vi "Test_API_InitInvalidInput_NoLogger.vi"(8 "error in (no error)":errorcluster, 11 "TestCase in":refnum<class "TestLocalLogInstance.lvclass">) -> (0 "error out":errorcluster, 3 "TestCase out":refnum<class "TestLocalLogInstance.lvclass">)   [LabVIEW 2017, in "TestLocalLogInstance.lvclass"]
uses:
  TestLocalLogInstance.lvclass
  Source/Composed Log/LoggerReference/LoggerReference.lvclass/LoggerReference.ctl
  9a0b009a-159a-478b-8bd0-efcaa49947a6.vi
  Source/Composed Log/LoggerReference/Return Aggregate Queues.vi
  Source/Composed Log/LoggerReference/Add Aggregate Log.vi
  9a0b009a-159a-478b-8bd0-efcaa49947a6.vi/c08b9aa3-6762-45d9-a18e-2ba9e4946dcb.vi
  Source/Composed Log/LoggerReference/Log.vi
  Source/Composed Log/LoggerReference/Send Add Sink.vi
  Source/Composed Log/LoggerReference/Remove Stale Logs.vi
  Source/Composed Log/Application Logger/Launch Worker Loop.vi
  Source/Composed Log/LoggerReference/Initialize Logger Instance.vi
  Source/Composed Log/Log Sink/Log Sink.lvclass
  Source/Composed Log/LoggerReference/LoggerReference.lvclass
  Source/Composed Log/IErrorFormat/IErrorFormat.lvclass
  <vilib>/addons/_JKI Toolkits/VI Tester/TestCase.llb/TestCase.lvclass
  C:/Program Files (x86)/National Instruments/LabVIEW 2017/vi.lib/addons/_JKI Toolkits/VI Tester/TestCase.llb/TestCase.lvclass
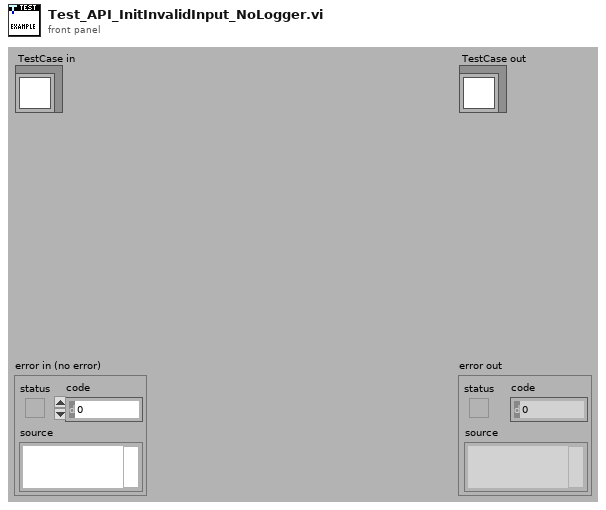
[diagram p1: front panel]
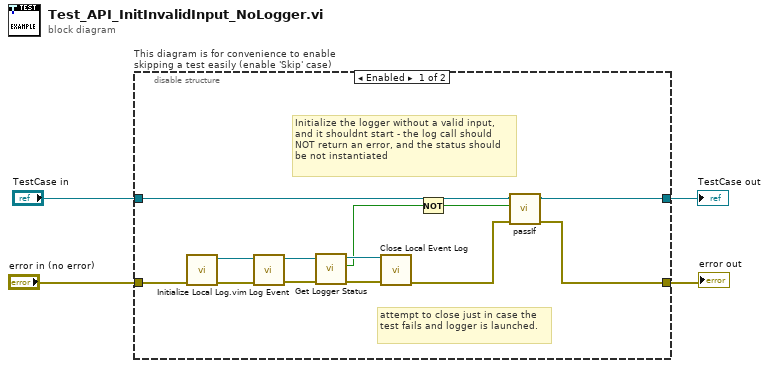
[diagram p0: block diagram]
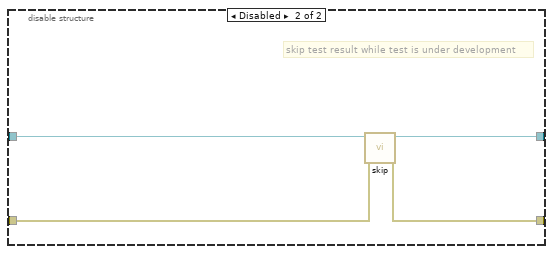
[diagram p2: hidden frame]
diagram:
  n1 = disable-structure "This diagram is for convenience to enable skipping a test easily (enable 'Skip' case)" shown="Enabled" {
    disable-tunnel: "TestCase in" -> [w14 w21]
    disable-tunnel: [w12 w19] -> w1
    disable-tunnel: [w11 w20] -> w3
    disable-tunnel: "error in (no error)" -> [w17 w18]
    frame Enabled {
      # "attempt to close just in case the test fails and logger is launched."
      # "Initialize the logger without a valid input, and it shouldnt start - the log call should  NOT return an error, and the status should be not instantiated"
      n2 = call "Initialize Local Log.vim"("error in (no error)"=w17) -> ("error out"=w16:errorcluster, "Log Instance Reference"=w15:refnum<class "LoggerReference.lvclass">)  [unwired: 8 in, 1 out]
      n3 = call "Log Event.vi"("error in (no error)"=w16, "Log Instance"=w15) -> ("error out"=w9:errorcluster, "Log Instance Out"=w10:refnum<class "LoggerReference.lvclass">)  [unwired: 8 in]
      n4 = call "Get Logger Status.vi"("error in (no error)"=w9, "LoggerReference in"=w10) -> ("error out"=w8:errorcluster, "Logger Instantiated?"=w6:bool, "LoggerReference out"=w7:refnum<class "LoggerReference.lvclass">)  [unwired: 6 in, 1 out]
      n5 = call "Close Local Event Log.vi"("error in (no error)"=w8, "Log Instance"=w7) -> ("error out"=w13:errorcluster)  [unwired: 9 in]
      n6 = Not(x=w6) -> (.not. x?=w5:bool)
      n7 = call-dynamic "passIf.vi"("error in (no error)"=w13, "pass"=w5, "TestCase in"=w14) -> ("error out"=w11:errorcluster, "TestCase out"=w12:refnum<class "TestLocalLogInstance.lvclass">)  [unwired: 7 in]
    }
    frame Disabled {
      # "skip test result while test is under development"
      n8 = call <vilib>:"skip.vi"("error in (no error)"=w18, "TestCase in"=w21) -> ("error out"=w20:errorcluster, "TestCase out"=w19:refnum<class "TestLocalLogInstance.lvclass">)  [unwired: 8 in]
    }
  }
  "error out" <- w3
  "TestCase out" <- w1
